vi "Close Instrument.vi"(8 "error in (no error)":errorcluster, 11 "instrument.PPMS2 in":refnum<class "instrument.PPMS.lvclass">) -> (0 "error out":errorcluster, 3 "instrument.PPMS2 out":refnum<class "instrument.PPMS.lvclass">)   [LabVIEW 2016, in "instrument.PPMS.lvclass"]
uses:
  instrument.PPMS.lvclass
  instrument.PPMS.lvclass/instrument.PPMS.ctl
  C:/user/patrick/hg/levylab_inst_ppms2/lvsrc/PPMS2/QDInstrument_LabView/QDInstrument.dll
  PPMS2/QDInstrument_LabView/QDInstrument.dll
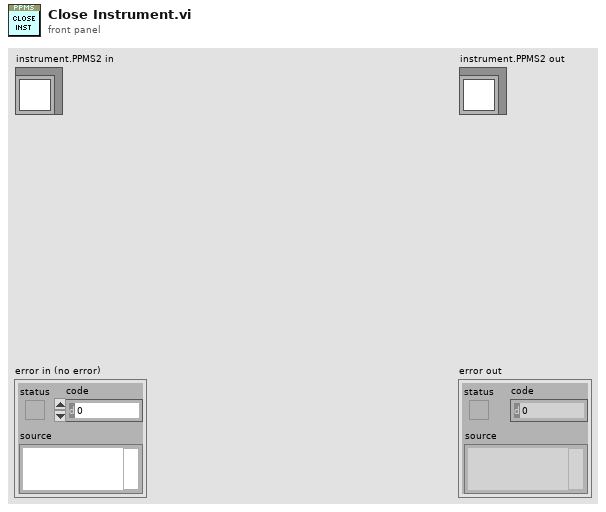
[diagram p1: front panel]
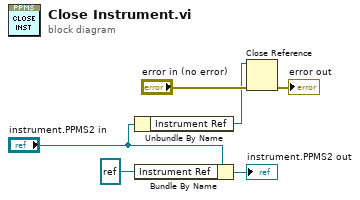
[diagram p0: block diagram]
diagram:
  n1 = Unbundle By Name("instrument.PPMS2 in") -> ("Instrument Ref"=w4:refnum<k24>)
  n2 = Bundle By Name(cluster="instrument.PPMS2 in", "Instrument Ref"=refnum<k24> refnum) -> (→"instrument.PPMS2 out":refnum<class "instrument.PPMS.lvclass">)
  n3 = Close Reference(reference=w4, error in (no error)="error in (no error)") -> (error out=→"error out":errorcluster)
